vi "SetupCallBackEvents.vi"(8 "error in (no error)":errorcluster, 11 "DataGridView in":refnum<class "DataGridView.lvclass">) -> (0 "error out":errorcluster, 3 "DataGridView out":refnum<class "DataGridView.lvclass">)   [LabVIEW 2016, in "DataGrid.lvlib" / "DataGridView.lvclass"]
doc: "Callbacks are used to tie the .net grid events to the labview event structure and this VI sets the callback VIs up for each of the possible events for the grid class."
uses:
  <userlib>/LabVIEWdotNetDataGrid/source/DataGridView/DataGridView.lvclass
  <userlib>/LabVIEWdotNetDataGrid/source/Events/Abstract EVENT/Abstract EVENT.lvclass
  <userlib>/LabVIEWdotNetDataGrid/source/DataGridView/DataGridView.lvclass/DataGridView.ctl
  <userlib>/LabVIEWdotNetDataGrid/source/DataGridView/Properties/Read DataGridView.vi
  System.Windows.Forms
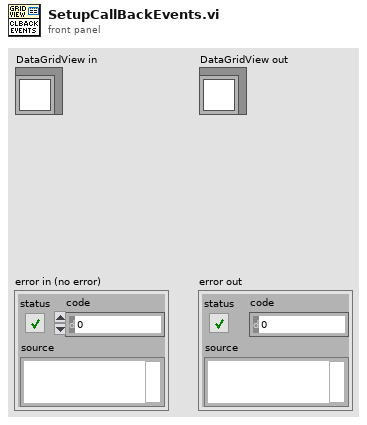
[diagram p1: front panel]
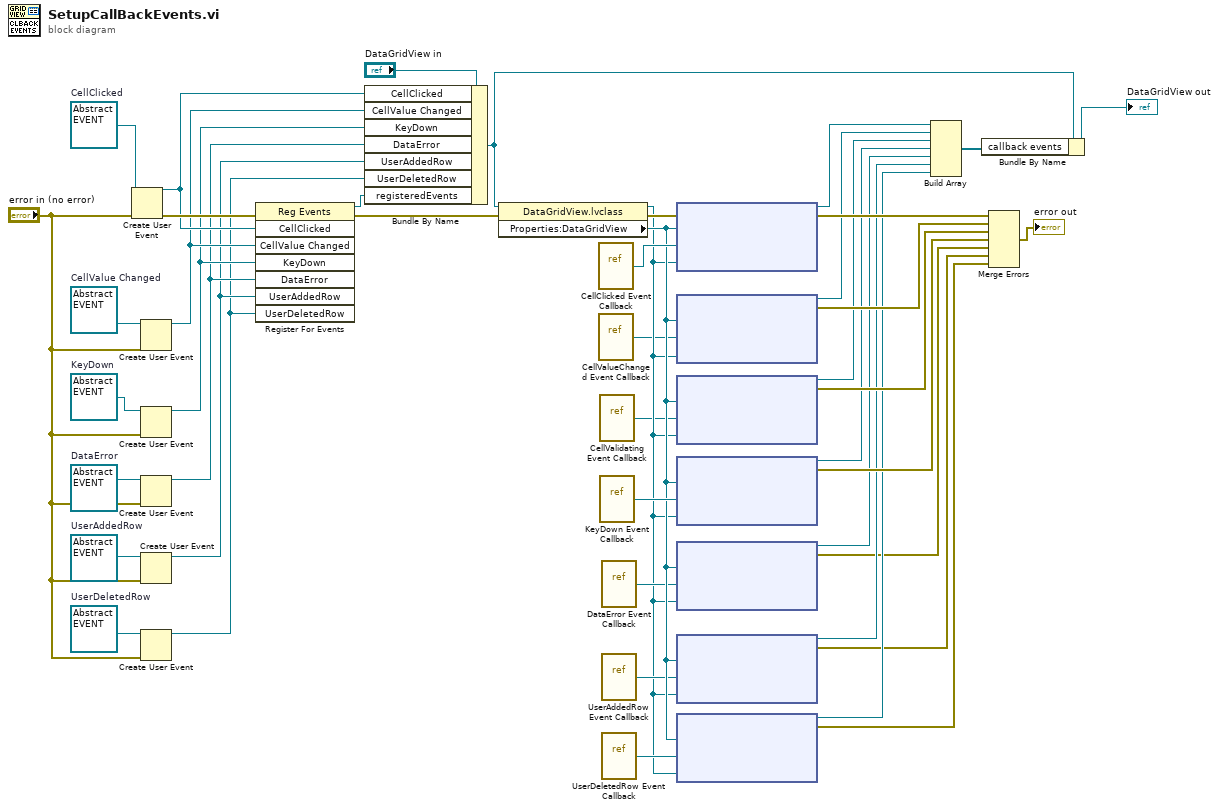
[diagram p0: block diagram]
diagram:
  w18 = refnum<class "Abstract EVENT.lvclass"> refnum  # UserDeletedRow
  w20 = refnum<class "Abstract EVENT.lvclass"> refnum  # UserAddedRow
  w19 = refnum<class "Abstract EVENT.lvclass"> refnum  # DataError
  w28 = refnum<class "Abstract EVENT.lvclass"> refnum  # KeyDown
  w32 = refnum<class "Abstract EVENT.lvclass"> refnum  # CellClicked
  w33 = refnum<class "Abstract EVENT.lvclass"> refnum  # CellValue Changed
  n1 = Create User Event(user event datatype=w32, error in="error in (no error)") -> (user event=w9:refnum<user-event>, error out=w45:errorcluster)
  n2 = Create User Event(user event datatype=w33, error in="error in (no error)") -> (user event=w8:refnum<user-event>)  [unwired: 1 out]
  n3 = Create User Event(user event datatype=w28, error in="error in (no error)") -> (user event=w7:refnum<user-event>)  [unwired: 1 out]
  n4 = Create User Event(user event datatype=w19, error in="error in (no error)") -> (user event=w6:refnum<user-event>)  [unwired: 1 out]
  n5 = Create User Event(user event datatype=w20, error in="error in (no error)") -> (user event=w5:refnum<user-event>)  [unwired: 1 out]
  n6 = Create User Event(user event datatype=w18, error in="error in (no error)") -> (user event=w4:refnum<user-event>)  [unwired: 1 out]
  n7 = register-events(error in=w45, w9, w8, w7, w6, w5, w4) -> (reference out=w2:refnum<event-registration>, error out=w43:errorcluster)  [unwired: 1 in]
  n8 = Bundle By Name(cluster="DataGridView in", "CellClicked"=w9, "CellValue Changed"=w8, "KeyDown"=w7, "DataError"=w6, "UserAddedRow"=w5, "UserDeletedRow"=w4, "registeredEvents"=w2) -> (w1:refnum<class "DataGridView.lvclass">)
  n9 = property class="DataGridView.lvclass"(reference=w1, error in=w43) -> (reference out=w22:refnum<class "DataGridView.lvclass">, error out=w44:errorcluster, "Properties:DataGridView"=w26:refnum<k24>)
  n10 = vi-ref <userlib>:"CellClicked Event Callback.vi"() -> ("vi reference"=w42:refnum<vi>)
  n11 = vi-ref <userlib>:"CellValueChanged Event Callback.vi"() -> ("vi reference"=w11:refnum<vi>)
  n12 = vi-ref <userlib>:"CellValidating Event Callback.vi"() -> ("vi reference"=w10:refnum<vi>)
  n13 = vi-ref <userlib>:"KeyDown Event Callback.vi"() -> ("vi reference"=w27:refnum<vi>)
  n14 = vi-ref <userlib>:"DataError Event Callback.vi"() -> ("vi reference"=w25:refnum<vi>)
  n15 = vi-ref <userlib>:"UserAddedRow Event Callback.vi"() -> ("vi reference"=w24:refnum<vi>)
  n16 = vi-ref <userlib>:"UserDeletedRow Event Callback.vi"() -> ("vi reference"=w23:refnum<vi>)
  n17 = node(w44, w26, w42, w22) -> (w37:refnum<k27>, w41:errorcluster)  [unwired: 1 in]
  n18 = node(w26, w11, w22) -> (w38:refnum<k27>, w40:errorcluster)  [unwired: 2 in]
  n19 = node(w26, w10, w22) -> (w36:refnum<k27>, w31:errorcluster)  [unwired: 2 in]
  n20 = node(w26, w27, w22) -> (w29:refnum<k27>, w30:errorcluster)  [unwired: 2 in]
  n21 = node(w26, w25, w22) -> (w17:refnum<k27>, w14:errorcluster)  [unwired: 2 in]
  n22 = node(w26, w24, w22) -> (w16:refnum<k27>, w13:errorcluster)  [unwired: 2 in]
  n23 = node(w26, w23, w22) -> (w15:refnum<k27>, w12:errorcluster)  [unwired: 2 in]
  n24 = Build Array(w37, w38, w36, w29, w17, w16, w15) -> (w34:refnum<k27>[])
  n25 = Bundle By Name(cluster=w1, "callback events"=w34) -> (→"DataGridView out":refnum<class "DataGridView.lvclass">)
  n26 = Merge Errors(w41, w40, w31, w30, w14, w13, w12) -> (→"error out":errorcluster)
